vi "CIF Manager UI.vi"() -> ()   [LabVIEW 2021, in "Inst Studio CIF Manager.lvlib"]
uses:
  Inst Studio CIF Manager.lvlib
  CIFPluginManager/gRPC/CIF_Manager_client/RPC Messages/cif_manager_PluginConfig.ctl
  PluginSDK/Plugin Events Enum.ctl
  CIFUI/CIF_UI.lvclass
  CIFUI/CIF_UI.lvclass/CIF_UI.ctl
  PluginSDK/Plugin Session.lvclass
  PluginSDK/InstrumentStudio Plugin SDK.lvlib
  CIFPluginManager/gRPC/CIF_Manager_Client_Wrapper/CIFManagerClientWrapper.lvlib
  <vilib>/gRPC/LabVIEW gRPC Library/grpc-lvsupport-release.lvlib
  CIFPluginManager/gRPC/CIF_Manager_client/CIF_Manager_client.lvlib
panel:
  in  "Tab Control 2":enum32{"System Monitoring", "Channels"}(tab)
  out "Connected":bool
  in  "Connect":bool
  in  "Running":bool
  in  "Loaded Plugins":string(tree)
  in  "Update Plugin Types":bool
  in  "Destroy":bool
  in  "stop":bool
  in  "Plugin Types":string(tree)
  in  "Get Loaded Plugins":bool
  in  "Load Plugin":bool
  in  "Plugin":T1
  in  "Abort Plugin":bool
  in  "plugin_name":string
  in  "Abort All Plugins":bool
  in  "address":string="192.168.1.160"
  in  "Errors":i32(listbox)=-1
  in  "Get Errors":bool
  in  "All Errors":bool
  in  "Reset Errors":bool
  out "local error":errorcluster
  in  "Clear Error":bool
  out "final errror":errorcluster
  out "Config":string
  in  "Reset Config":bool
  in  "All Config":bool
  in  "Get Config":bool
  in  "Reset Info":bool
  out "Info":string
  in  "All Info":bool
  in  "Get Info":bool
  out "Server dll path":path
  out "Event Record":i32(listbox)
  in  "Session Id":u64
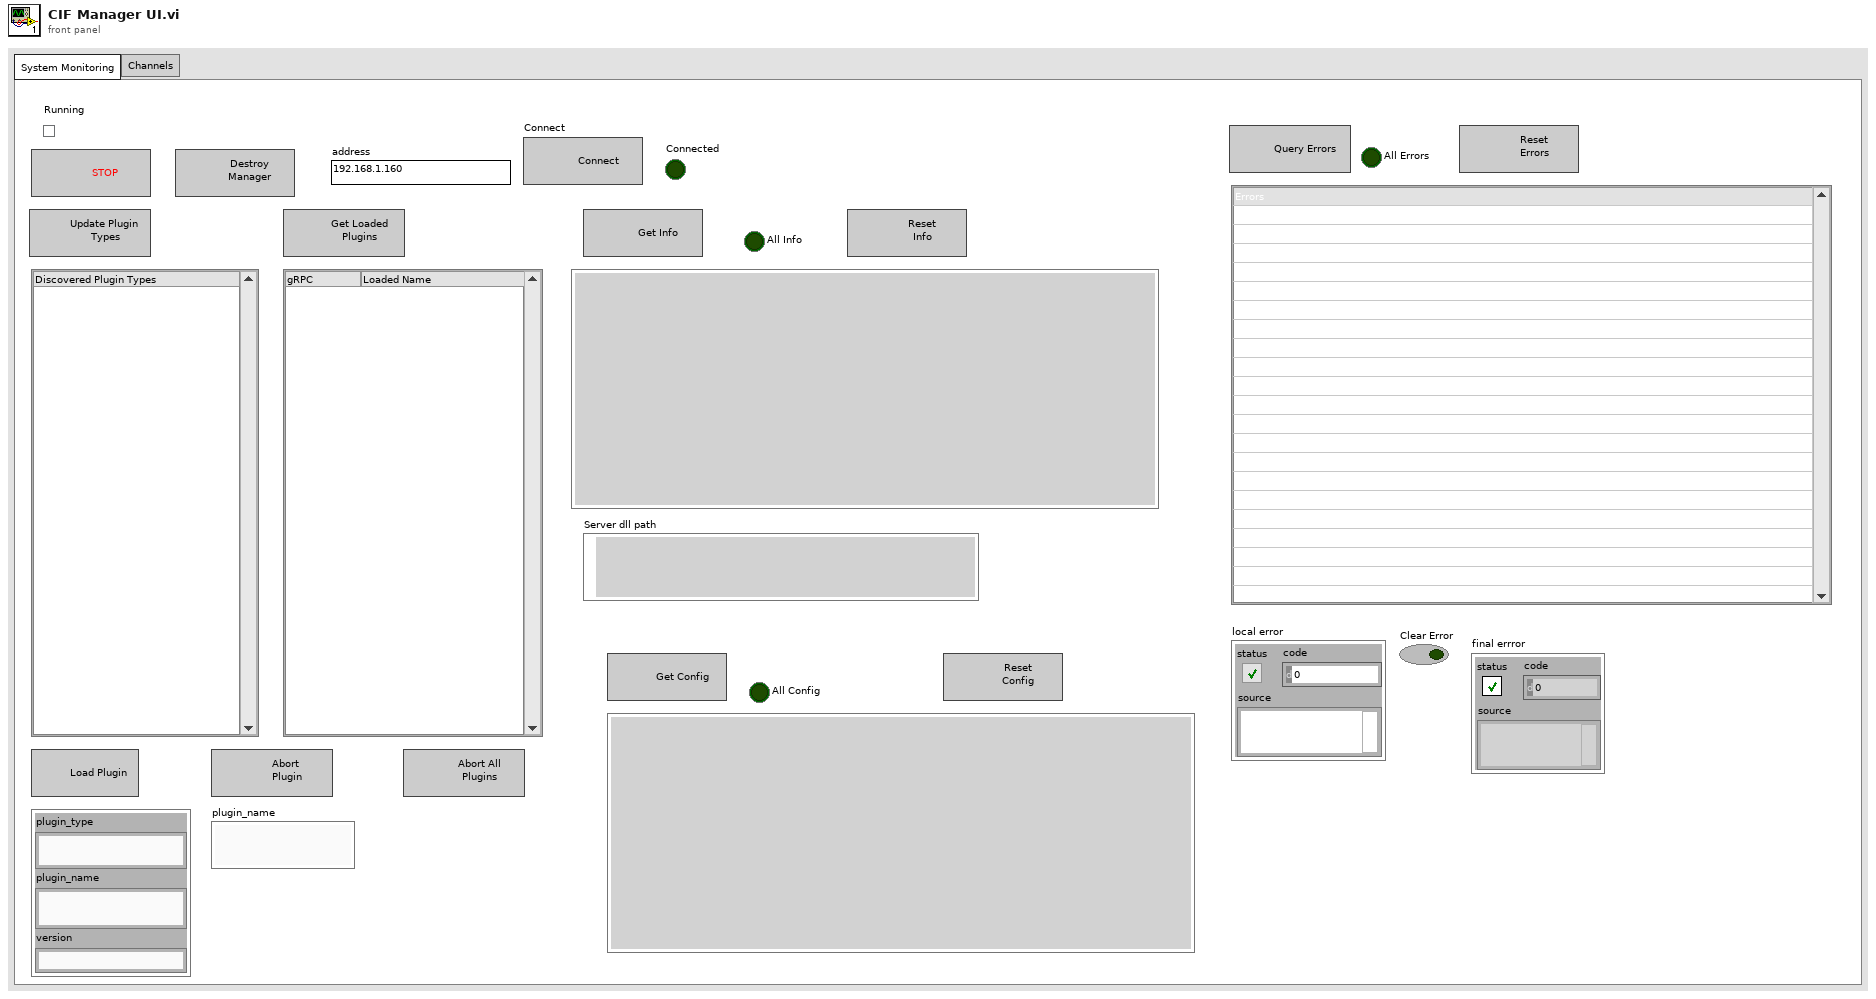
[diagram p1: front panel]
types:
  T1 = typedef "CIF_Manager_client.lvlib/cif_manager_PluginConfig.ctl" = cluster{"plugin_type":string, "plugin_name":string, "version":string}
  T2 = typedef "InstrumentStudio Plugin SDK.lvlib/Plugin Events Enum.ctl" = enum32{"Shutdown", "Project Saved", "Stop All Outputs", "Generic Message", "Active Pin Map Changed", "Selected Sites Changed"}
  T3 = typedef "InstrumentStudio Plugin SDK.lvlib/Event Registration Refnum.ctl" = refnum<event-registration>
  T4 = typedef "grpc-lvsupport-release.lvlib/grpcId.ctl" = u64
  T5 = typedef "CIF_Manager_client.lvlib/cif_manager_PluginType.ctl" = cluster{"plugin_type":string, "plugin_version":T6}
  T6 = typedef "CIF_Manager_client.lvlib/cif_manager_PluginVersion.ctl" = cluster{"major_version":i32, "minor_version":i32, "fix_version":i32, "build_version":i32}
  T7 = typedef "CIF_Manager_client.lvlib/cif_manager_PluginInfo.ctl" = cluster{"plugin_name":string, "plugin_type":string, "grpc_port":i32, "plugin_version":T6, "status":T8}
  T8 = typedef "CIF_Manager_client.lvlib/cif_plugincore_StatusData.ctl" = cluster{"state":T9, "timing_statistics":T10, "fifo_statistics":T12, "error":T13, "monitor_doubles":T14, "monitor_u64s":T15, "monitor_i64s":T16}
  T9 = typedef "CIF_Manager_client.lvlib/cif_plugincore_StatusData_State.ctl" = enum32{"NULL", "CREATING", "LISTENING", "RUNNING", "CLEANINGUP", "DESTROYING"}
  T10 = typedef "CIF_Manager_client.lvlib/cif_plugincore_TimingStatistics.ctl" = cluster{"period":T11, "wake_error":T11, "execute":T11, "housekeep":T11, "idle":T11}
  T11 = typedef "CIF_Manager_client.lvlib/cif_plugincore_TimingStatsBasic.ctl" = cluster{"max":i32, "min":i32}
  T12 = typedef "CIF_Manager_client.lvlib/cif_plugincore_FifoStatistics.ctl" = cluster{"from_t0":T11, "from_previous_plugin":T11, "output_error":T11}
  T13 = typedef "CIF_Manager_client.lvlib/cif_plugincore_Error.ctl" = cluster{"status":bool, "code":i32}
  T14 = typedef "CIF_Manager_client.lvlib/cif_plugincore_MonitorDoubles.ctl" = cluster{"double_1":dbl, "double_2":dbl, "double_3":dbl, "double_4":dbl}
  T15 = typedef "CIF_Manager_client.lvlib/cif_plugincore_MonitorU64.ctl" = cluster{"u64_1":u64, "u64_2":u64, "u64_3":u64, "u64_4":u64}
  T16 = typedef "CIF_Manager_client.lvlib/cif_plugincore_MonitorI64.ctl" = cluster{"i64_1":i64, "i64_2":i64, "i64_3":i64, "i64_4":i64}
  T17 = typedef "CIF_Manager_client.lvlib/cif_manager_ErrorInfo.ctl" = cluster{"error_status":bool, "error_code":i32, "plugin":string, "time":string, "message":string, "location":string}
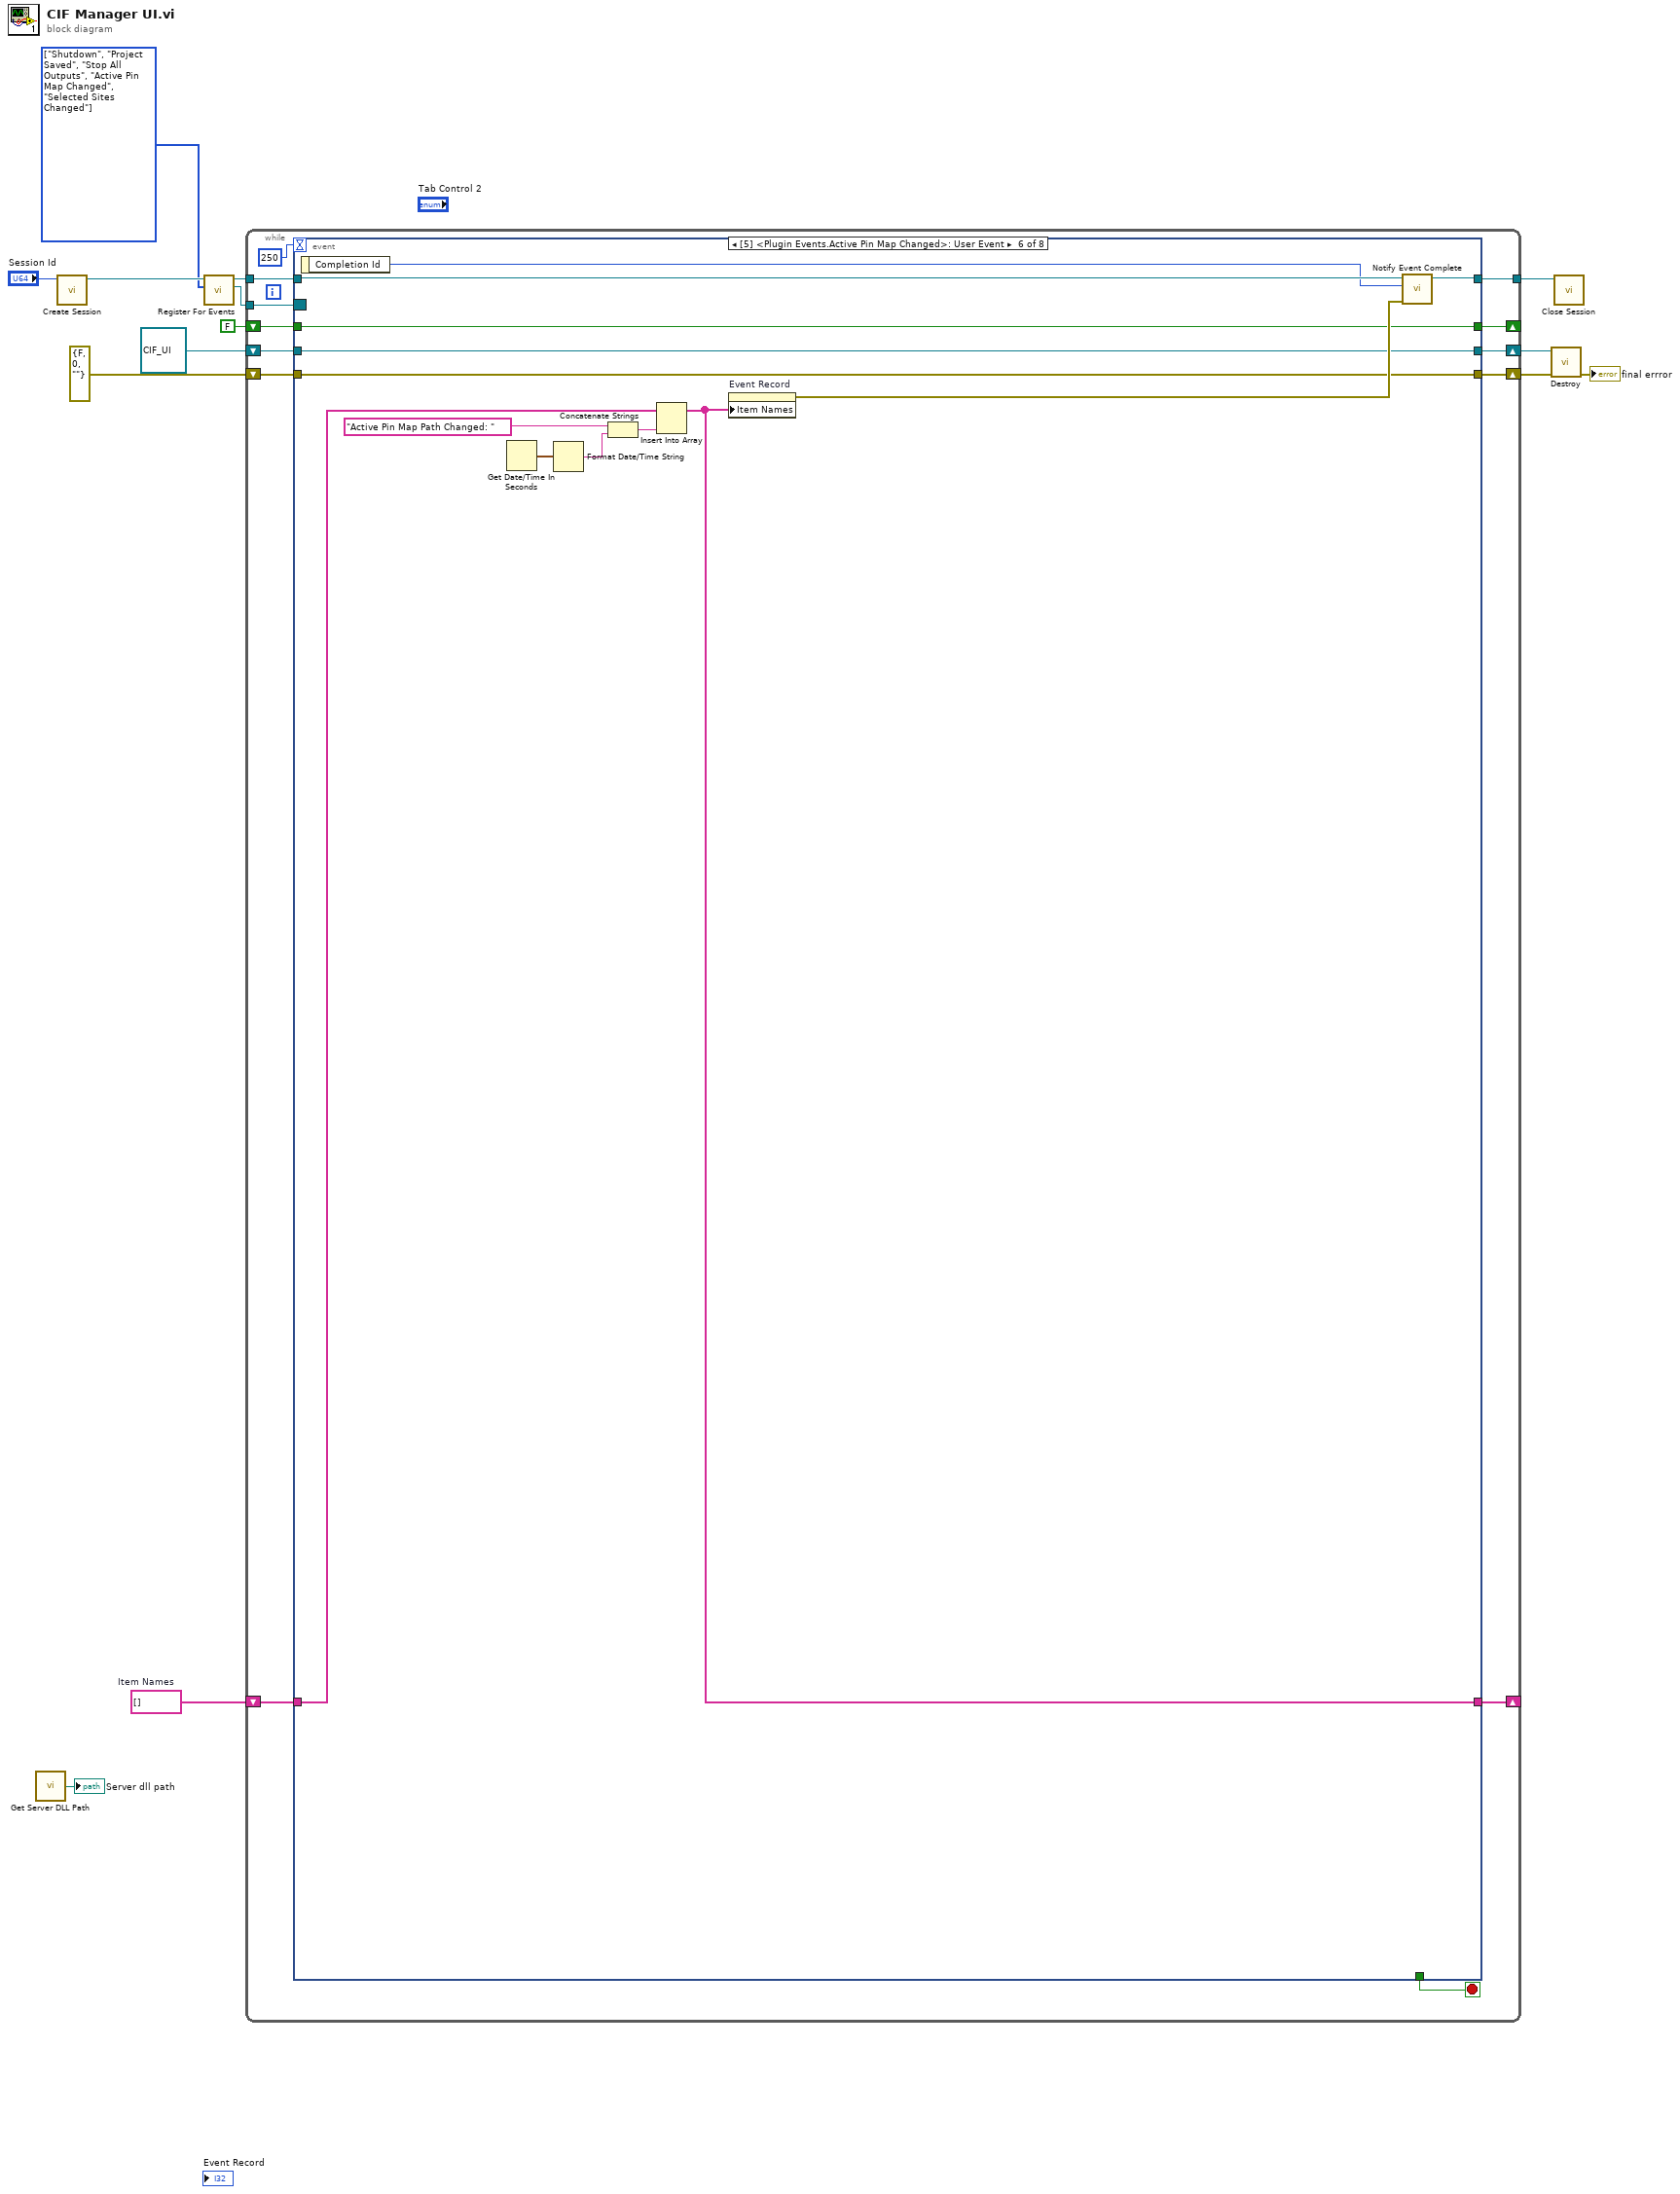
[diagram p0: block diagram]
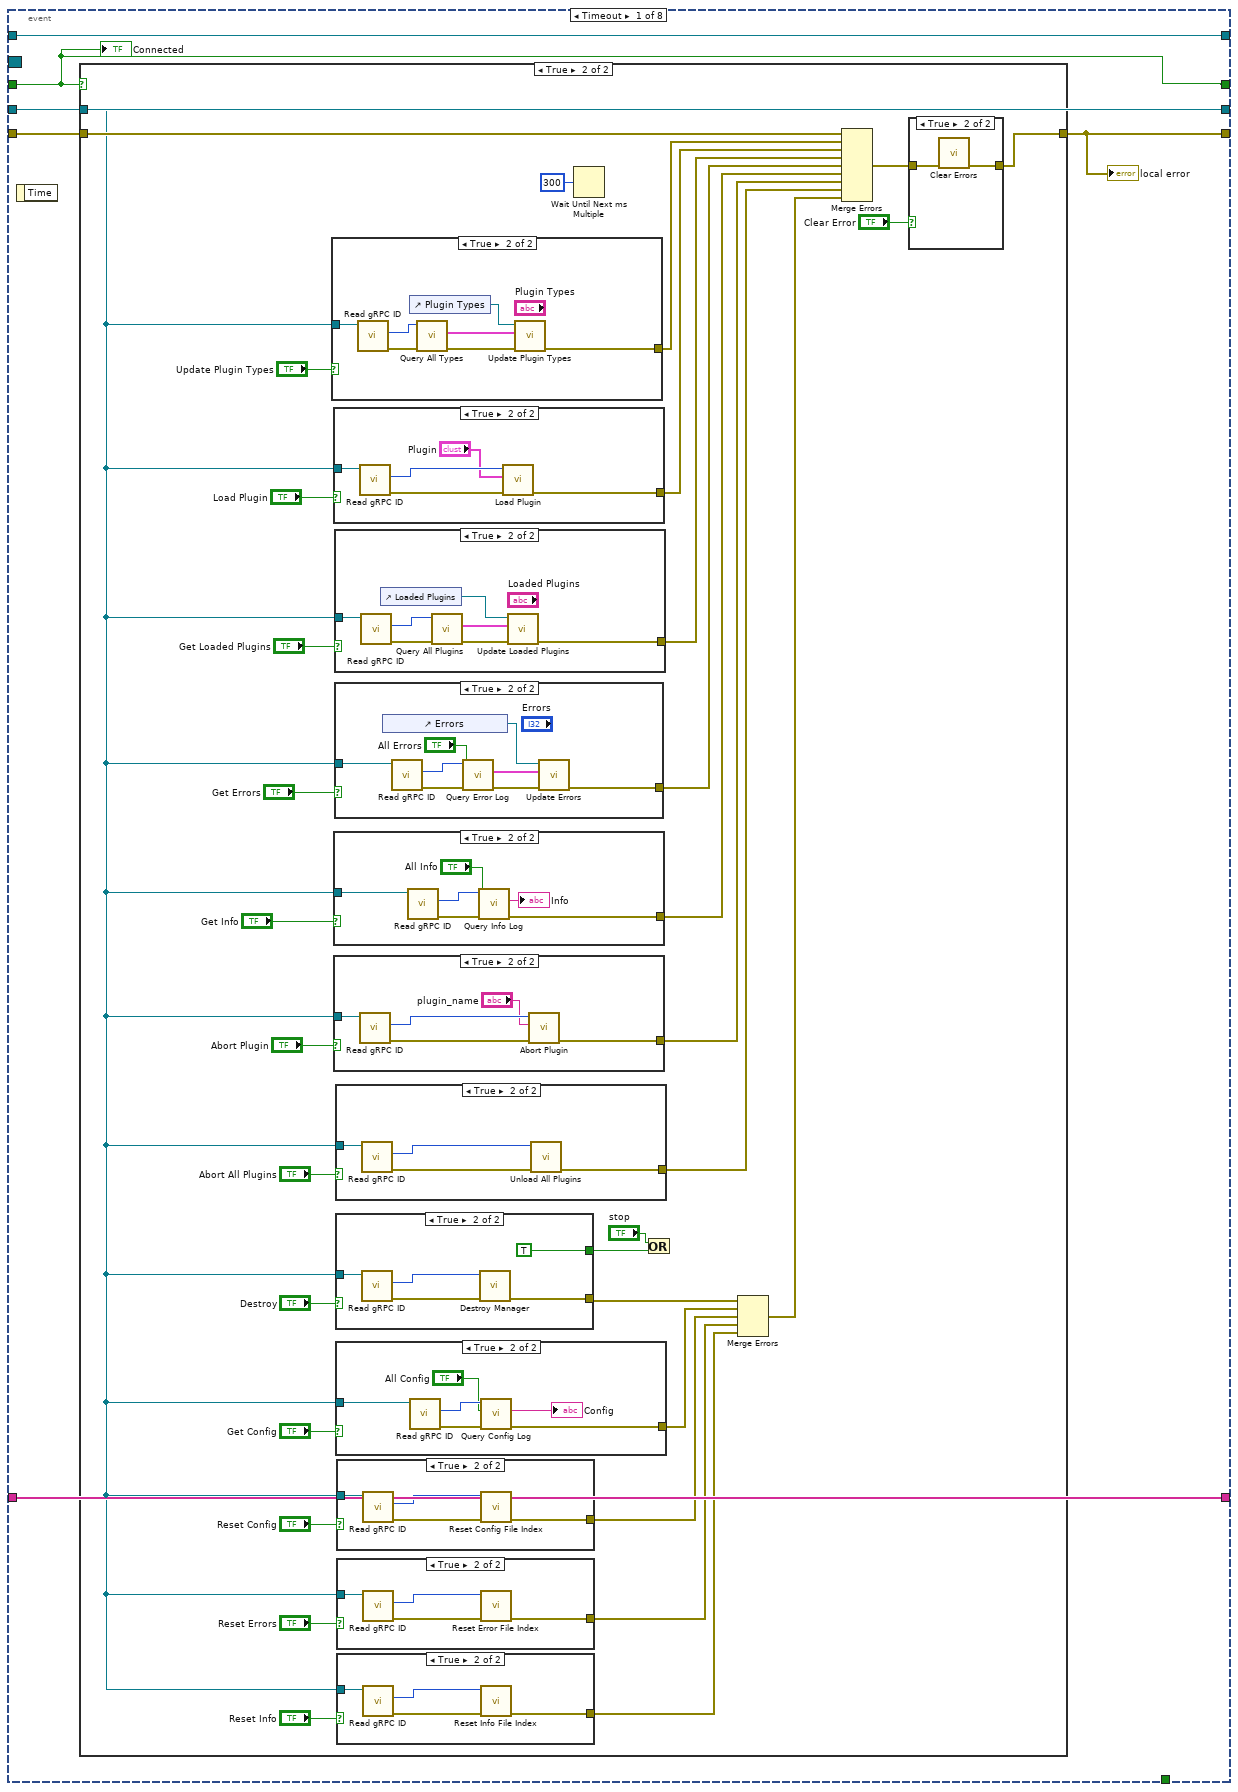
[diagram p2: hidden frame]
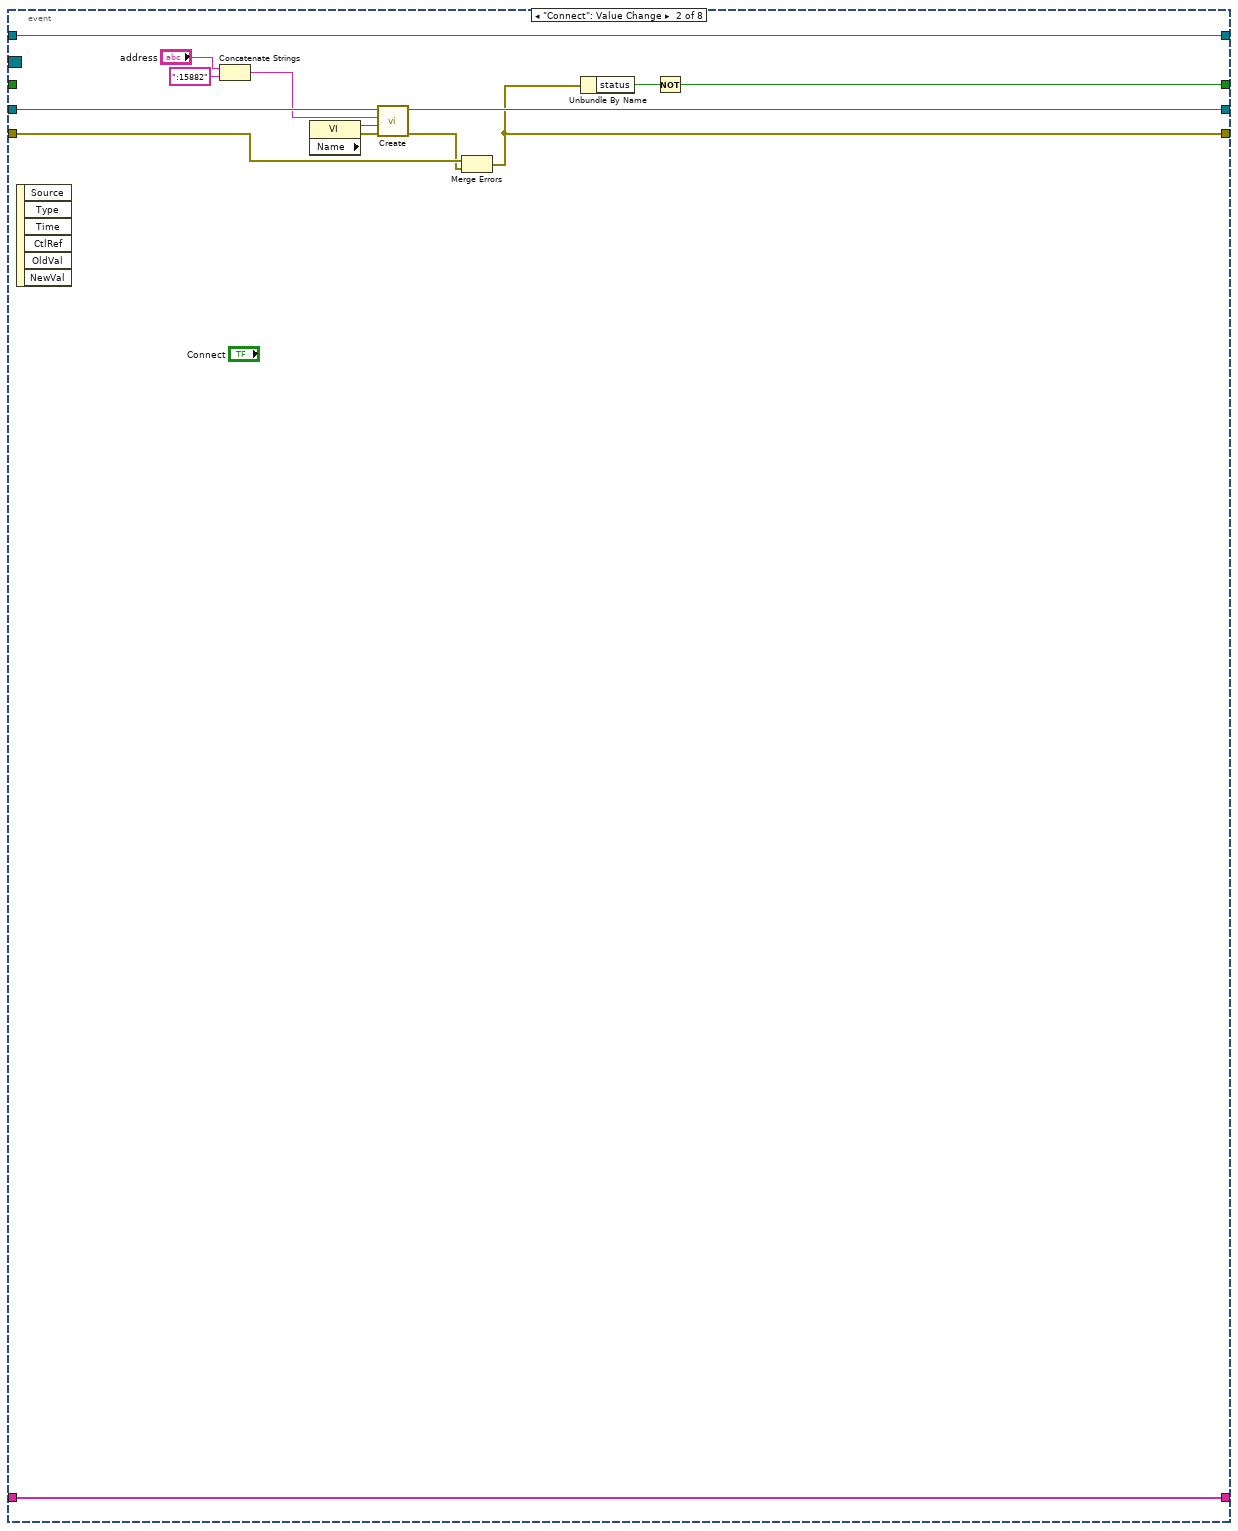
[diagram p17: hidden frame]
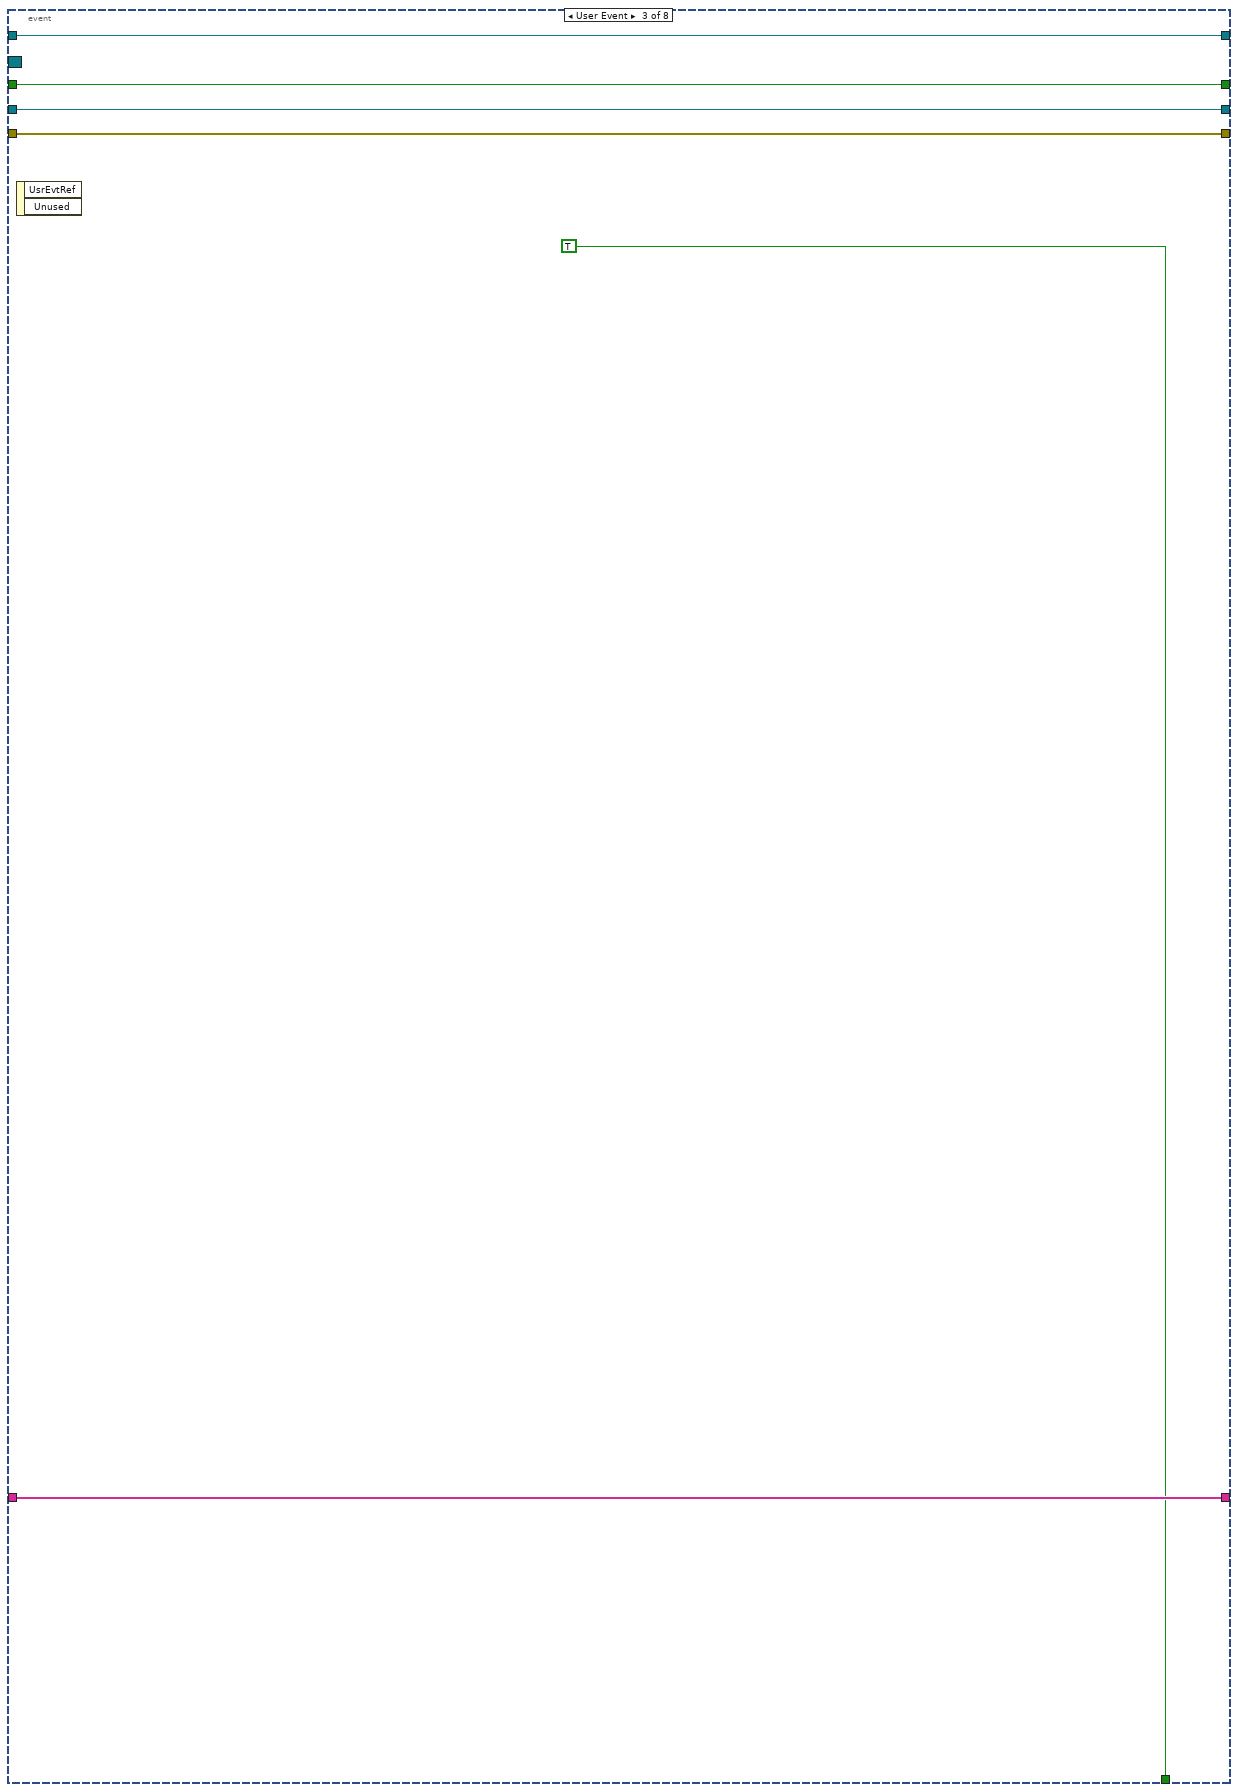
[diagram p18: hidden frame]
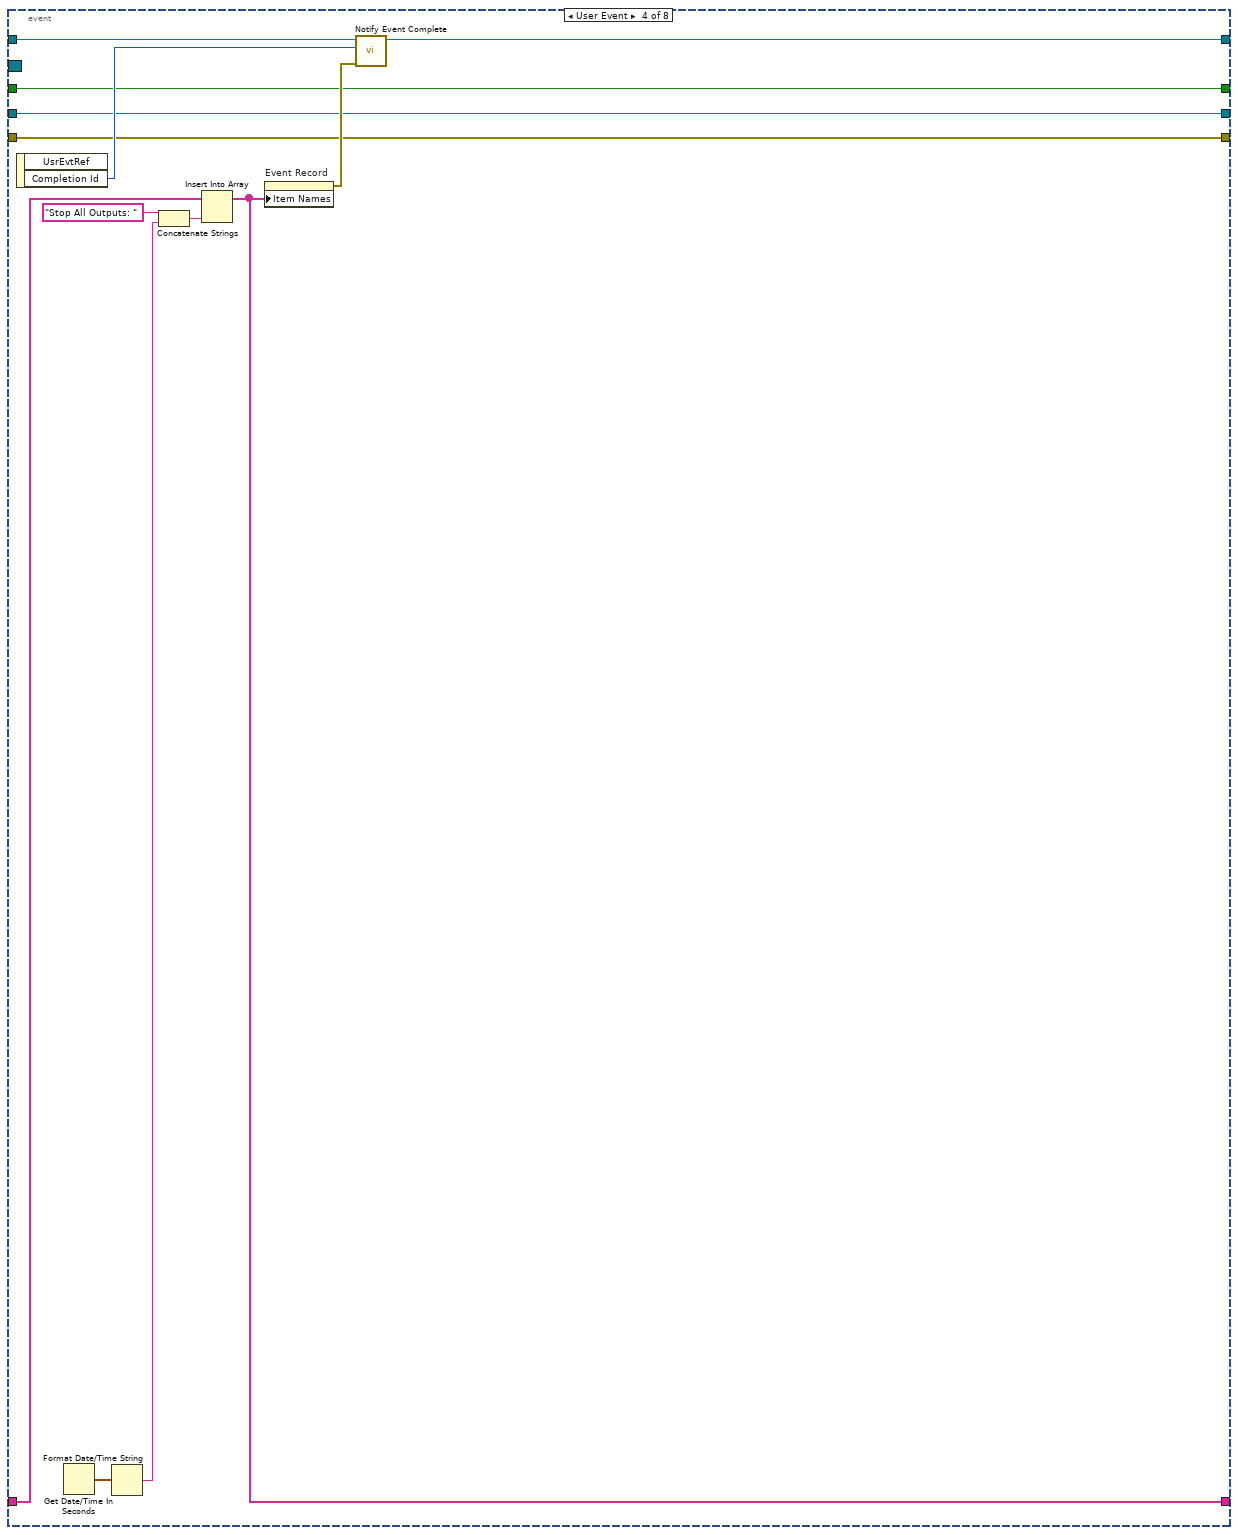
[diagram p19: hidden frame]
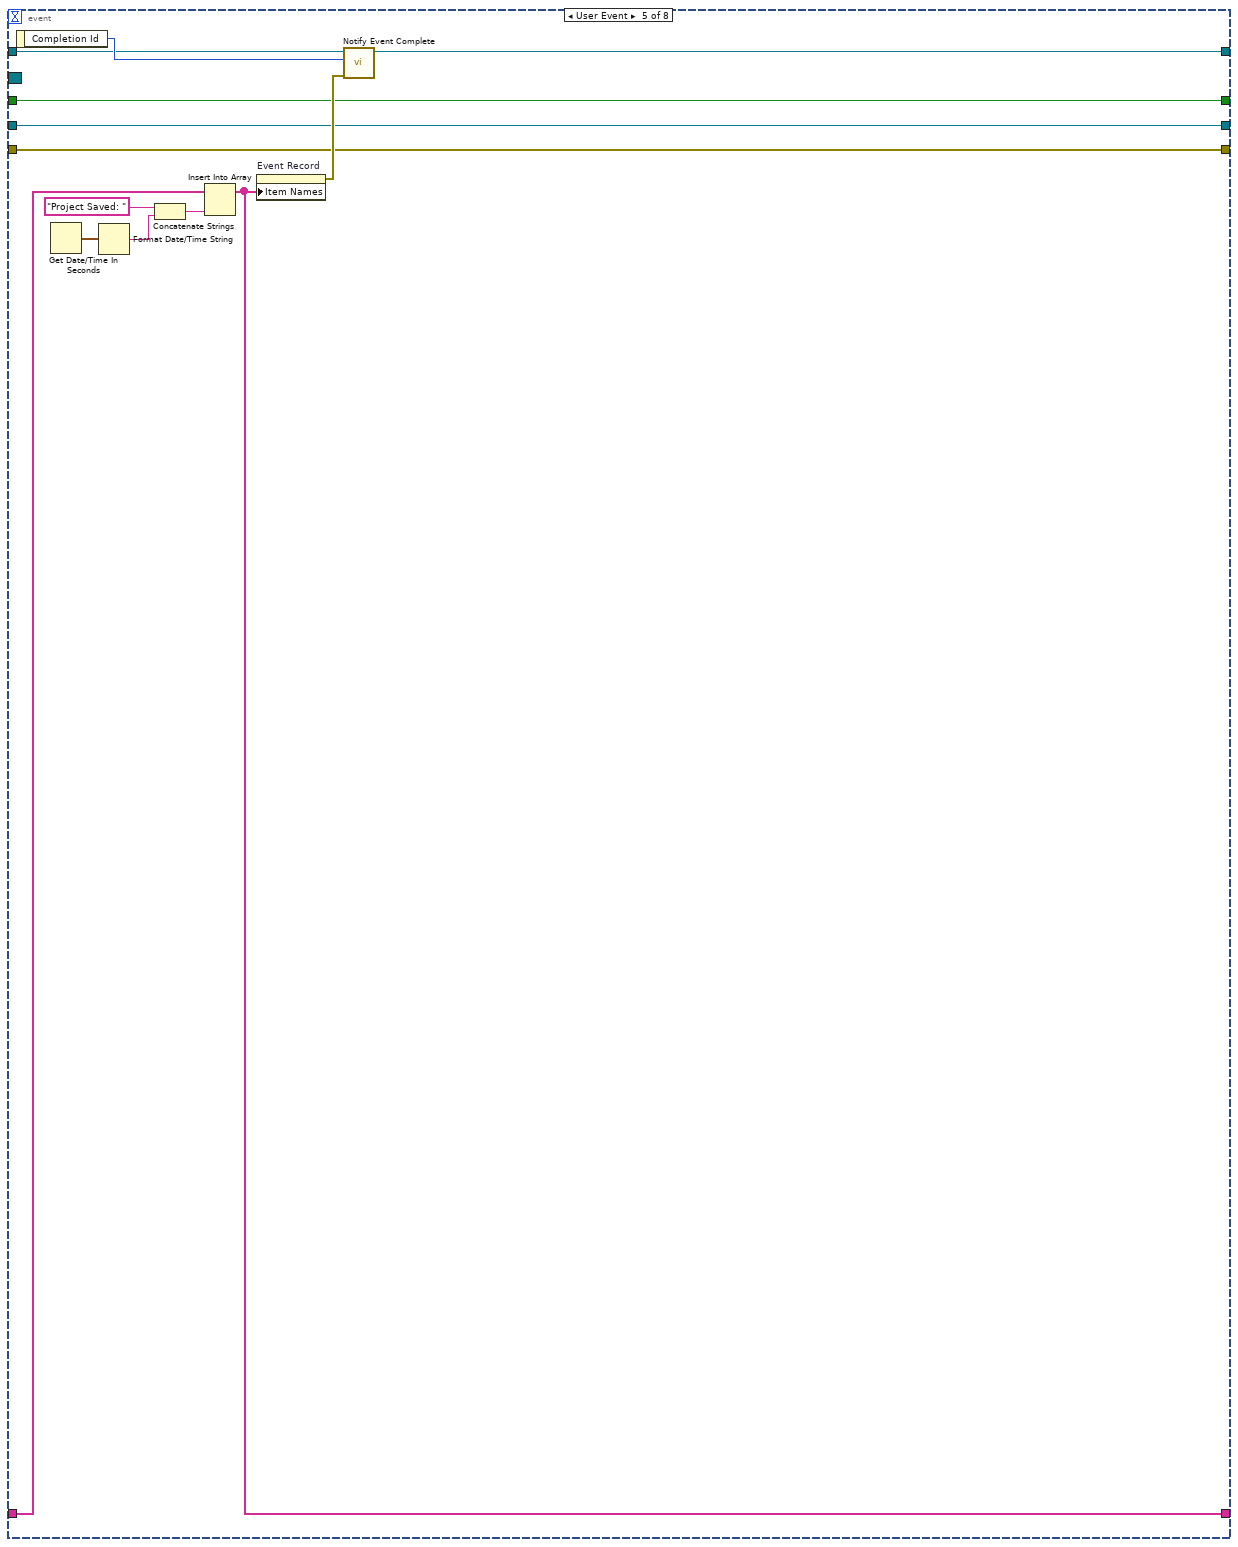
[diagram p20: hidden frame]
diagram:
  w9 = T2[] [enum."Shutdown", enum."Project Saved", enum."Stop All Outputs", enum."Active Pin Map Changed", enum."Selected Sites Changed"] items=["Shutdown", "Project Saved", "Stop All Outputs", "Generic Message", "Active Pin Map Changed", "Selected Sites Changed"] ("Events To Register")
  w12 = string[] []  # Item Names
  n1 = call <vilib>:"Get Server DLL Path.vi"() -> ("Server dll path"=→"Server dll path":path)
  n2 = call "Create Session.vi"("Session Id"="Session Id") -> ("Session out"=w13:refnum<class "Plugin Session.lvclass">)  [unwired: 6 in, 4 out]
  n3 = call "Register For Events.vi"("Events To Register"=w9, "Session in"=w13) -> ("Event Refnum"=w8:T3, "Session out"=w11:refnum<class "Plugin Session.lvclass">)  [unwired: 7 in, 1 out]
  n4 = while {
    shift-right: [w25] -> _
    shift-left: w12 -> [w26]
    tunnel: w11 -> [w24]
    tunnel: [w23] -> w10
    tunnel: w8 -> [w22]
    shift-right: [w17] -> w5
    shift-left: refnum<class "CIF_UI.lvclass"> refnum ("CIF_UI out") -> [w20]
    shift-right: [w15] -> _
    shift-left: FALSE -> [w16]
    shift-right: [w18] -> w6
    shift-left: errorcluster {"status"=FALSE, "code"=0, "source"=""} ("error out") -> [w19]
    stop <- w21 stop-if-true
    n5 = event shown="[5] <Plugin Events.Active Pin Map Changed>: User Event" {
      selector: w22 -> [_ _ _ _ _ _ _ _]
      dyn-events: _ -> [_ _ _ _ _ _ _ _]
      timeout: 250 -> [_ _ _ _ _ _ _ _]
      tunnel: w26 -> [w33 w149 w155 w164 w180 w189 w203 w214]
      tunnel: [w33 w149 w155 w163 w176 w188 w202 w214] -> w25
      tunnel: w24 -> [w32 w136 w153 w162 w174 w187 w200 w213]
      tunnel: [w32 w136 w153 w161 w173 w186 w201 w212] -> w23
      tunnel: [_ _ TRUE _ _ _ _ _] -> w21
      tunnel: w20 -> [w30 w146 w152 w157 w170 w184 w196 w209]
      tunnel: w19 -> [w31 w141 w151 w158 w169 w183 w195 w208]
      tunnel: [w29 w139 w151 w158 w169 w183 w195 w208] -> w18
      tunnel: [w30 w142 w152 w157 w170 w184 w196 w209] -> w17
      tunnel: w16 -> [w28 _ w150 w156 w171 w182 w197 w210]
      tunnel: [w28 w137 w150 w156 w171 w182 w197 w210] -> w15
      event Timeout {
        n6 = event-data() -> ()  [unwired: 1 in, 1 out]
        n7 = case shown="True" w28 {
          tunnel: w31 -> [w34 w67]
          tunnel: [w34 w66] -> w29
          tunnel: w30 -> [_ w65]
          frame False {
          }
          frame True {
            n8 = case shown="True" "Update Plugin Types" {
              tunnel: w65 -> [_ w135]
              tunnel: [_ w129] -> w64
              frame False {
              }
              frame True {
                n9 = call "Read gRPC ID.vi"("CIF_UI in"=w135) -> ("error out"=w130:errorcluster, "gRPCid"=w131:T4)  [unwired: 8 in, 1 out]
                n10 = control-ref of="Plugin Types"() -> (w133:refnum<vi>)
                n11 = call "Query All Types.vi"("error in"=w130, "gRPC ID in"=w131) -> ("error out"=w134:errorcluster, "plugin_types"=w132:T5[])  [unwired: 7 in, 1 out]
                n12 = call "Update Plugin Types.vi"("error in (no error)"=w134, "plugin_types"=w132, "Plugin Types ref in"=w133) -> ("error out"=w129:errorcluster)  [unwired: 7 in, 1 out]
              }
            }
            n13 = case shown="True" "Load Plugin" {
              tunnel: w65 -> [_ w125]
              tunnel: [_ w122] -> w59
              frame False {
              }
              frame True {
                n14 = call "Read gRPC ID.vi"("CIF_UI in"=w125) -> ("error out"=w123:errorcluster, "gRPCid"=w124:T4)  [unwired: 8 in, 1 out]
                n15 = call "Load Plugin.vi"("error in"=w123, "Plugin"="Plugin", "gRPC ID in"=w124) -> ("error out"=w122:errorcluster)  [unwired: 7 in, 1 out]
              }
            }
            n16 = case shown="True" "Get Info" {
              tunnel: w65 -> [_ w105]
              tunnel: [_ w102] -> w56
              frame False {
              }
              frame True {
                n17 = call "Read gRPC ID.vi"("CIF_UI in"=w105) -> ("error out"=w103:errorcluster, "gRPCid"=w104:T4)  [unwired: 8 in, 1 out]
                n18 = call "Query Info Log.vi"("error in"=w103, "query_all"="All Info", "gRPC ID in"=w104) -> ("error out"=w102:errorcluster, "Info"=→"Info":string)  [unwired: 6 in, 1 out]
              }
            }
            n19 = case shown="True" "Abort Plugin" {
              tunnel: w65 -> [_ w99]
              tunnel: [_ w96] -> w55
              frame False {
              }
              frame True {
                n20 = call "Read gRPC ID.vi"("CIF_UI in"=w99) -> ("error out"=w97:errorcluster, "gRPCid"=w98:T4)  [unwired: 8 in, 1 out]
                n21 = call "Abort Plugin.vi"("error in"=w97, "plugin_name"="plugin_name", "gRPC ID in"=w98) -> ("error out"=w96:errorcluster)  [unwired: 7 in, 1 out]
              }
            }
            n22 = case shown="True" "Get Loaded Plugins" {
              tunnel: w65 -> [_ w120]
              tunnel: [_ w114] -> w58
              frame False {
              }
              frame True {
                n23 = call "Read gRPC ID.vi"("CIF_UI in"=w120) -> ("error out"=w118:errorcluster, "gRPCid"=w119:T4)  [unwired: 8 in, 1 out]
                n24 = control-ref of="Loaded Plugins"() -> (w115:refnum<vi>)
                n25 = call "Query All Plugins.vi"("error in"=w118, "gRPC ID in"=w119) -> ("error out"=w116:errorcluster, "plugin_info"=w117:T7[])  [unwired: 7 in, 1 out]
                n26 = call "Update Loaded Plugins.vi"("error in (no error)"=w116, "plugin_info"=w117, "Loaded Plugins ref in"=w115) -> ("error out"=w114:errorcluster)  [unwired: 7 in, 1 out]
              }
            }
            n27 = case shown="True" "Get Errors" {
              tunnel: w65 -> [_ w113]
              tunnel: [_ w106] -> w57
              frame False {
              }
              frame True {
                n28 = control-ref of="Errors"() -> (w107:refnum<vi>)
                n29 = call "Read gRPC ID.vi"("CIF_UI in"=w113) -> ("error out"=w111:errorcluster, "gRPCid"=w112:T4)  [unwired: 8 in, 1 out]
                n30 = call "Query Error Log.vi"("error in"=w111, "query_all"="All Errors", "gRPC ID in"=w112) -> ("error out"=w109:errorcluster, "error_info"=w108:T17[])  [unwired: 6 in, 1 out]
                n31 = call "Update Errors.vi"("error in (no error)"=w109, "error_info"=w108, "Error MCLB reference in"=w107) -> ("error out"=w106:errorcluster)  [unwired: 7 in, 1 out]
              }
            }
            n32 = case shown="True" "Abort All Plugins" {
              tunnel: w65 -> [_ w94]
              tunnel: [_ w91] -> w54
              frame False {
              }
              frame True {
                n33 = call "Read gRPC ID.vi"("CIF_UI in"=w94) -> ("error out"=w92:errorcluster, "gRPCid"=w93:T4)  [unwired: 8 in, 1 out]
                n34 = call "Unload All Plugins.vi"("error in"=w92, "gRPC ID in"=w93) -> ("error out"=w91:errorcluster)  [unwired: 8 in, 1 out]
              }
            }
            n35 = case shown="True" "Destroy" {
              tunnel: w65 -> [_ w90]
              tunnel: [_ w87] -> w43
              tunnel: [_ TRUE] -> w46
              frame False {
              }
              frame True {
                n36 = call "Read gRPC ID.vi"("CIF_UI in"=w90) -> ("error out"=w88:errorcluster, "gRPCid"=w89:T4)  [unwired: 8 in, 1 out]
                n37 = call "Destroy Manager.vi"("error in"=w88, "gRPC ID in"=w89) -> ("error out"=w87:errorcluster)  [unwired: 8 in, 1 out]
              }
            }
            n38 = case shown="True" "Get Config" {
              tunnel: w65 -> [_ w85]
              tunnel: [_ w82] -> w41
              frame False {
              }
              frame True {
                n39 = call "Read gRPC ID.vi"("CIF_UI in"=w85) -> ("error out"=w83:errorcluster, "gRPCid"=w84:T4)  [unwired: 8 in, 1 out]
                n40 = call "Query Config Log.vi"("error in"=w83, "query_all"="All Config", "gRPC ID in"=w84) -> ("error out"=w82:errorcluster, "Config"=→"Config":string)  [unwired: 6 in, 1 out]
              }
            }
            n41 = case shown="True" "Reset Config" {
              tunnel: w65 -> [_ w79]
              tunnel: [_ w76] -> w40
              frame False {
              }
              frame True {
                n42 = call "Read gRPC ID.vi"("CIF_UI in"=w79) -> ("error out"=w77:errorcluster, "gRPCid"=w78:T4)  [unwired: 8 in, 1 out]
                n43 = call "Reset Config File Index.vi"("error in"=w77, "gRPC ID in"=w78) -> ("error out"=w76:errorcluster)  [unwired: 8 in, 1 out]
              }
            }
            n44 = case shown="True" "Reset Errors" {
              tunnel: w65 -> [_ w75]
              tunnel: [_ w72] -> w36
              frame False {
              }
              frame True {
                n45 = call "Read gRPC ID.vi"("CIF_UI in"=w75) -> ("error out"=w73:errorcluster, "gRPCid"=w74:T4)  [unwired: 8 in, 1 out]
                n46 = call "Reset Error File Index.vi"("error in"=w73, "gRPC ID in"=w74) -> ("error out"=w72:errorcluster)  [unwired: 8 in, 1 out]
              }
            }
            n47 = case shown="True" "Reset Info" {
              tunnel: w65 -> [_ w71]
              tunnel: [_ w68] -> w35
              frame False {
              }
              frame True {
                n48 = call "Read gRPC ID.vi"("CIF_UI in"=w71) -> ("error out"=w69:errorcluster, "gRPCid"=w70:T4)  [unwired: 8 in, 1 out]
                n49 = call "Reset Info File Index.vi"("error in"=w69, "gRPC ID in"=w70) -> ("error out"=w68:errorcluster)  [unwired: 8 in, 1 out]
              }
            }
            n50 = Wait Until Next ms Multiple(millisecond multiple=u32 300) -> ()  [unwired: 1 out]
            n51 = Or(x="stop", y=w46) -> ()  [unwired: 1 out]
            n52 = Merge Errors(w43, w41, w40, w36, w35) -> (w44:errorcluster)
            n53 = Merge Errors(w67, w64, w59, w58, w57, w56, w55, w54, w44) -> (w62:errorcluster)
            n54 = case shown="True" "Clear Error" {
              tunnel: w62 -> [w126 w128]
              tunnel: [w126 w127] -> w66
              frame False {
              }
              frame True {
                n55 = call <vilib>:"Clear Errors.vi"("error in (no error)"=w128) -> ("error out"=w127:errorcluster)  [unwired: 5 in, 1 out]
              }
            }
          }
        }
        "local error" <- w29
        "Connected" <- w28
      }
      event "Connect": Value Change {
        n56 = event-data() -> ()  [unwired: 1 in, 6 out]
        n57 = Concatenate Strings("address", ":15882" ("string")) -> (w143:string)
        n58 = property class="VI" props=["Name"]() -> (reference out=w148:refnum<vi>, error out=w147:errorcluster)  [unwired: 2 in, 1 out]
        n59 = call "Create.vi"("error in (no error)"=w147, "VI Reference"=w148, "Manager Address"=w143, "CIF_UI in"=w146) -> ("error out"=w140:errorcluster, "CIF_UI out"=w142:refnum<class "CIF_UI.lvclass">)  [unwired: 6 in]
        n60 = Merge Errors(w141, w140) -> (w139:errorcluster)
        n61 = Unbundle By Name(w139) -> ("status"=w138:bool)
        n62 = Not(x=w138) -> (.not. x?=w137:bool)
      }
      event User Event {
        n63 = event-data() -> ()  [unwired: 1 in, 2 out]
      }
      event User Event {
        n64 = event-data() -> ("Completion Id"=w160:i64)  [unwired: 1 in, 1 out]
        n65 = Get Date/Time In Seconds() -> (seconds since 1Jan1904=w165:timestamp)
        n66 = Format Date/Time String(seconds (now)=w165) -> (date/time string=w167:string)  [unwired: 2 in]
        n67 = Concatenate Strings("Stop All Outputs: ", w167) -> (w166:string)
        n68 = Insert Into Array(array=w164, new element=w166) -> (w163:string[])  [unwired: 1 in]
        n69 = property on="Event Record" class="LstBox (strict)"("Item Names"=w163) -> (error out=w159:errorcluster)  [unwired: 2 in, 1 out]
        n70 = call "Notify Event Complete.vi"("error in (no error)"=w159, "Completion Id"=w160, "Session in"=w162) -> ("Session out"=w161:refnum<class "Plugin Session.lvclass">)  [unwired: 7 in, 1 out]
      }
      event User Event {
        n71 = event-data() -> ("Completion Id"=w181:i64)  [unwired: 1 in]
        n72 = Get Date/Time In Seconds() -> (seconds since 1Jan1904=w175:timestamp)
        n73 = Format Date/Time String(seconds (now)=w175) -> (date/time string=w178:string)  [unwired: 2 in]
        n74 = Concatenate Strings("Project Saved: ", w178) -> (w177:string)
        n75 = Insert Into Array(array=w180, new element=w177) -> (w176:string[])  [unwired: 1 in]
        n76 = property on="Event Record" class="LstBox (strict)"("Item Names"=w176) -> (error out=w172:errorcluster)  [unwired: 2 in, 1 out]
        n77 = call "Notify Event Complete.vi"("error in (no error)"=w172, "Completion Id"=w181, "Session in"=w174) -> ("Session out"=w173:refnum<class "Plugin Session.lvclass">)  [unwired: 7 in, 1 out]
      }
      event User Event {
        n78 = event-data() -> ("Completion Id"=w185:i64)  [unwired: 1 in]
        n79 = Get Date/Time In Seconds() -> (seconds since 1Jan1904=w191:timestamp)
        n80 = Format Date/Time String(seconds (now)=w191) -> (date/time string=w193:string)  [unwired: 2 in]
        n81 = Concatenate Strings("Active Pin Map Path Changed: ", w193) -> (w192:string)
        n82 = Insert Into Array(array=w189, new element=w192) -> (w188:string[])  [unwired: 1 in]
        n83 = property on="Event Record" class="LstBox (strict)"("Item Names"=w188) -> (error out=w190:errorcluster)  [unwired: 2 in, 1 out]
        n84 = call "Notify Event Complete.vi"("error in (no error)"=w190, "Completion Id"=w185, "Session in"=w187) -> ("Session out"=w186:refnum<class "Plugin Session.lvclass">)  [unwired: 7 in, 1 out]
      }
      event User Event {
        n85 = event-data() -> ("Completion Id"=w198:i64)  [unwired: 1 in]
        n86 = Get Date/Time In Seconds() -> (seconds since 1Jan1904=w204:timestamp)
        n87 = Format Date/Time String(seconds (now)=w204) -> (date/time string=w206:string)  [unwired: 2 in]
        n88 = Concatenate Strings("Selected Sites Changed: ", w206) -> (w205:string)
        n89 = Insert Into Array(array=w203, new element=w205) -> (w202:string[])  [unwired: 1 in]
        n90 = property on="Event Record" class="LstBox (strict)"("Item Names"=w202) -> (error out=w199:errorcluster)  [unwired: 2 in, 1 out]
        n91 = call "Notify Event Complete.vi"("error in (no error)"=w199, "Completion Id"=w198, "Session in"=w200) -> ("Session out"=w201:refnum<class "Plugin Session.lvclass">)  [unwired: 7 in, 1 out]
      }
      event "Running": Value Change {
        n92 = event-data() -> ()  [unwired: 1 in, 5 out]
        n93 = call "Update Running State.vi"("Is Running"="Running", "Plugin Session in"=w213) -> ("Plugin Session out"=w212:refnum<class "Plugin Session.lvclass">)  [unwired: 8 in, 1 out]
      }
    }
  }
  n94 = call "Destroy.vi"("error in (no error)"=w6, "CIF_UI in"=w5) -> ("error out"=→"final errror":errorcluster)  [unwired: 8 in, 1 out]
  n95 = call "Close Session.vi"("Session in"=w10) -> ()  [unwired: 10 in, 1 out]
